vi "2019-05-14_Variable.vi"() -> ()   [LabVIEW 2018]
panel:
  in  "정지 버튼":bool
  out "웨이브폼 차트 3":dbl(graph)
  out "웨이브폼 차트 2":dbl(graph)
  out "웨이브폼 차트":dbl(graph)
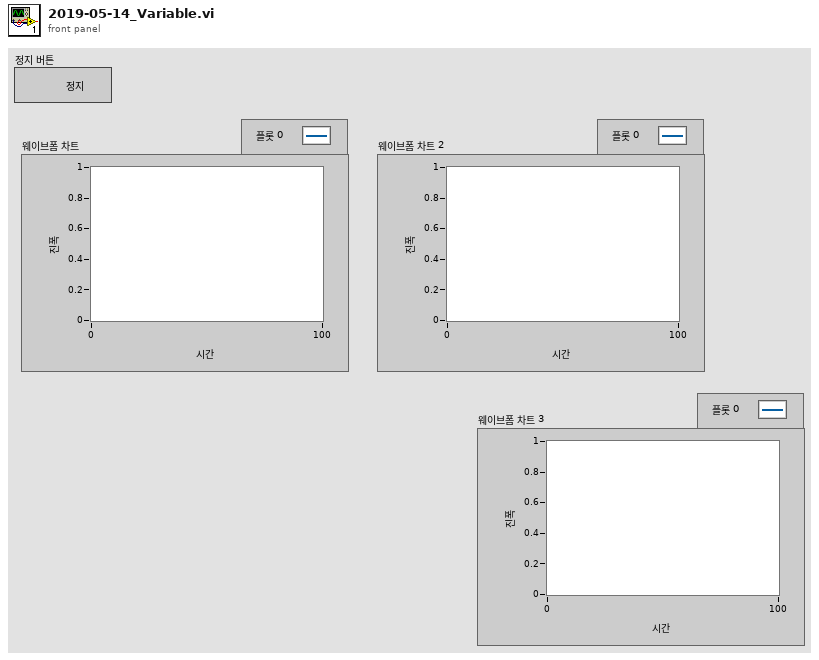
[diagram p1: front panel]
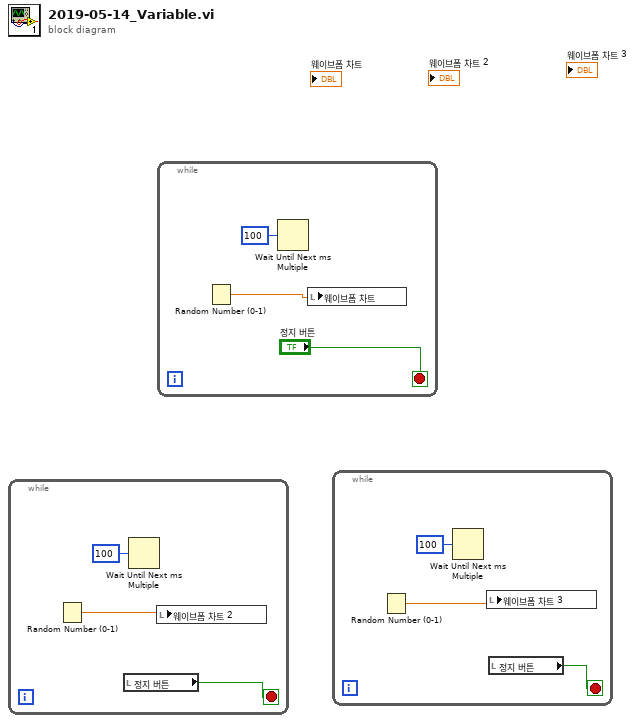
[diagram p0: block diagram]
diagram:
  n1 = while {
    stop <- w1 stop-if-true
    n2 = Random Number (0-1)() -> (number: 0 to 1=w2:dbl)
    n3 = local read "정지 버튼"() -> (w1:bool)
    n4 = Wait Until Next ms Multiple(millisecond multiple=u32 100 ("ms 배수")) -> ()  [unwired: 1 out]
    n5 = local write "웨이브폼 차트 2"(w2) -> ()
  }
  n6 = while {
    stop <- "정지 버튼" stop-if-true
    n7 = Random Number (0-1)() -> (number: 0 to 1=w5:dbl)
    n8 = Wait Until Next ms Multiple(millisecond multiple=u32 100 ("ms 배수")) -> ()  [unwired: 1 out]
    n9 = local write "웨이브폼 차트"(w5) -> ()
  }
  n10 = while {
    stop <- w7 stop-if-true
    n11 = Random Number (0-1)() -> (number: 0 to 1=w8:dbl)
    n12 = Wait Until Next ms Multiple(millisecond multiple=u32 100 ("ms 배수")) -> ()  [unwired: 1 out]
    n13 = local write "웨이브폼 차트 3"(w8) -> ()
    n14 = local read "정지 버튼"() -> (w7:bool)
  }
